vi "Calculate Maximum from Segment.vi"(9 "Sample Number":dbl, 10 "Begin Sample":dbl, 11 "Dynamic Data Type":dynamicdata(waveform)) -> (2 "Section":dynamicdata(waveform), 3 "Peak Force":dbl)   [LabVIEW 2016]
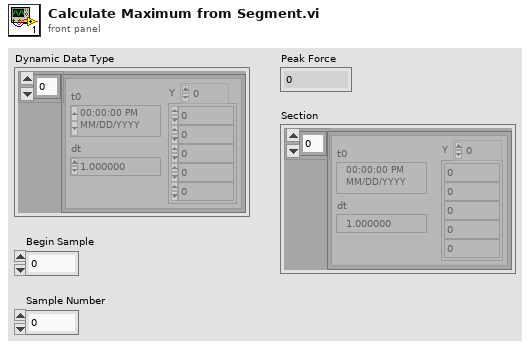
[diagram p1: front panel]
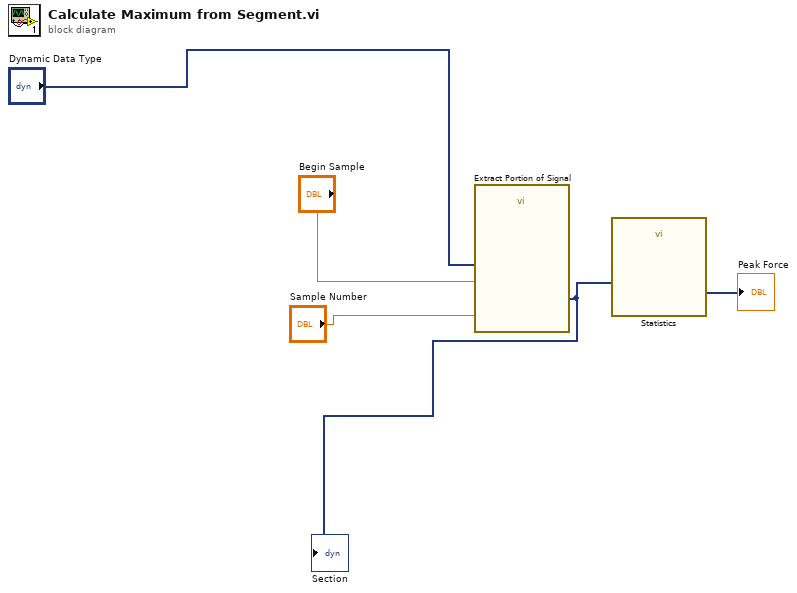
[diagram p0: block diagram]
diagram:
  n1 = call "Extract Portion of Signal"("Samples"="Sample Number", "Begin Sample"="Begin Sample", "Signals"="Dynamic Data Type") -> ("Section"=w5:dynamicdata)  [unwired: 7 in, 1 out]
  "Section" <- w5
  n2 = call "Statistics"("Signals"=w5) -> ("Maximum"=→"Peak Force":dynamicdata)  [unwired: 25 in, 1 out]
